vi "tx Rx Packet.vi"(10 "protocol_version":i32, 11 "port_num":i32) -> ()   [LabVIEW 2021, in "dxl_x86_c.lvlib"]
doc: "WINDECLSPEC void txRxPacket (int port_num, int protocol_version);"
uses:
  dxl_x86_c.lvlib
  dxl_x86_c.dll
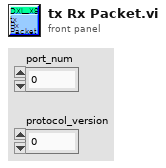
[diagram p1: front panel]
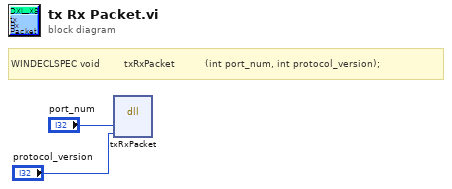
[diagram p0: block diagram]
diagram:
  # "WINDECLSPEC void        txRxPacket          (int port_num, int protocol_version);"
  n1 = dll-call lib="C:/Users/ashek/Desktop/ashekim/ws/DynamixelSDK/labview/labview/dxl_x86_c.*" fn="txRxPacket"("port_num"="port_num", "protocol_version"="protocol_version") -> ()  [unwired: 6 in, 2 out]
